vi "Read Shared Variables - SuNLaMP DO.vi"(9 "channel errors in (no errors)":errorcluster[](array[cluster])) -> (1 "channel errors out":errorcluster[](array[cluster]), 2 "data":dbl[](array[numeric]), 3 "UUIDs":string[](array[string])=["Flow Rate [g/s]", "Density [g/cm^3]", "Return Filter dP [psid]", "Outlet Filter and Flowmeter dp [psid]", "Cooler dP [psid]", "Cooler CO2 In [F]", "Cooler CO2 Out [F]", "Pump Frequency [%]", "Recirc Valve Open [%]"])   [LabVIEW 2020]
uses:
  <vilib>/Utility/error.llb/Error Cluster From Error Code.vi
  <vilib>/ErrorRing/Error Ring.xnode
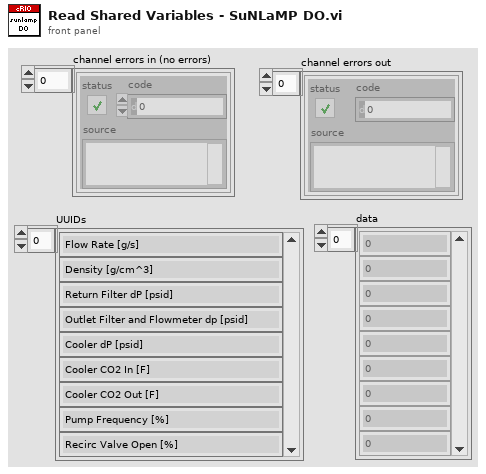
[diagram p1: front panel]
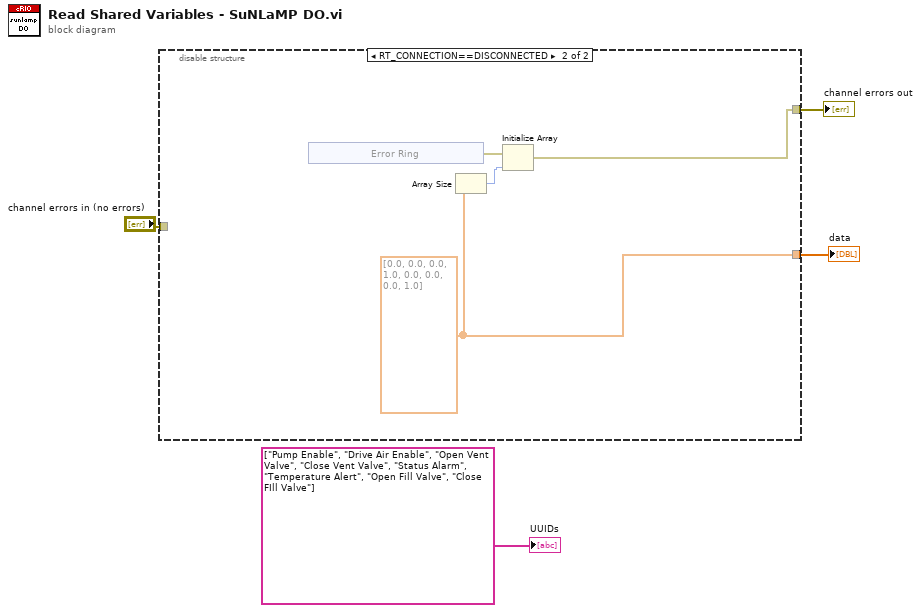
[diagram p0: block diagram]
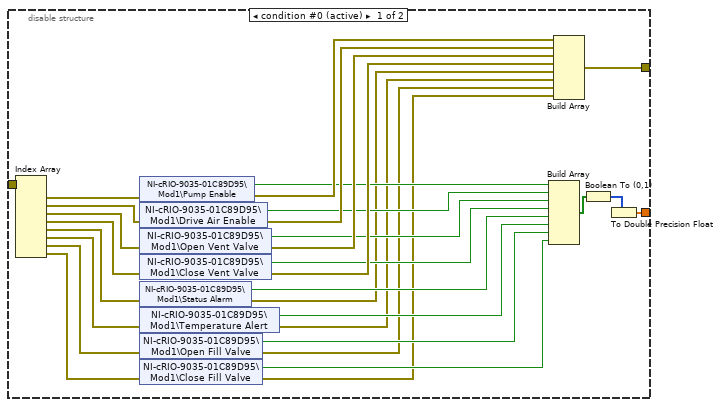
[diagram p2: hidden frame]
diagram:
  n1 = disable-structure shown="RT_CONNECTION==DISCONNECTED" {
    disable-tunnel: [w24 w35] -> w3
    disable-tunnel: "channel errors in (no errors)" -> [w23 _]
    disable-tunnel: [w17 w34] -> w1
    frame condition #0 (active) {
      n2 = Index Array(array=w23) -> (element #1=w22:errorcluster, element #2=w21:errorcluster, element #3=w20:errorcluster, element #4=w19:errorcluster, element #5=w16:errorcluster, element #6=w15:errorcluster, element #7=w14:errorcluster, element #8=w13:errorcluster)  [unwired: 8 in]
      n3 = shared-variable "NI-cRIO-9035-01C89D95\\Mod1\\Pump Enable"(error in=w22) -> (w26:bool, error out=w30:errorcluster)
      n4 = shared-variable "NI-cRIO-9035-01C89D95\\Mod1\\Drive Air Enable"(error in=w21) -> (w27:bool, error out=w31:errorcluster)
      n5 = shared-variable "NI-cRIO-9035-01C89D95\\Mod1\\Open Vent Valve"(error in=w20) -> (w28:bool, error out=w32:errorcluster)
      n6 = shared-variable "NI-cRIO-9035-01C89D95\\Mod1\\Close Vent Valve"(error in=w19) -> (w29:bool, error out=w33:errorcluster)
      n7 = shared-variable "NI-cRIO-9035-01C89D95\\Mod1\\Status Alarm"(error in=w16) -> (w12:bool, error out=w8:errorcluster)
      n8 = shared-variable "NI-cRIO-9035-01C89D95\\Mod1\\Temperature Alert"(error in=w15) -> (w11:bool, error out=w7:errorcluster)
      n9 = shared-variable "NI-cRIO-9035-01C89D95\\Mod1\\Open Fill Valve"(error in=w14) -> (w10:bool, error out=w6:errorcluster)
      n10 = shared-variable "NI-cRIO-9035-01C89D95\\Mod1\\Close Fill Valve"(error in=w13) -> (w9:bool, error out=w5:errorcluster)
      n11 = Build Array(w26, w27, w28, w29, w12, w11, w10, w9) -> (w25:bool[])
      n12 = Build Array(w30, w31, w32, w33, w8, w7, w6, w5) -> (w24:errorcluster[])
      n13 = Boolean To (0,1)(Boolean=w25) -> (0, 1=w18:i16[])
      n14 = To Double Precision Float(number=w18) -> (double precision float=w17:dbl[])
    }
    frame condition #1 {
      w34 = dbl[] [0.0, 0.0, 0.0, 1.0, 0.0, 0.0, 0.0, 1.0] ("data")
      n15 = xnode "Error Ring"() -> ("error out"=w37:errorcluster)
      n16 = Array Size(array=w34) -> (size(s)=w36:i32)
      n17 = Initialize Array(w37, w36) -> (w35:errorcluster[])
    }
  }
  "data" <- w1
  "channel errors out" <- w3
  "UUIDs" <- string[] ["Pump Enable", "Drive Air Enable", "Open Vent Valve", "Close Vent Valve", "Status Alarm", "Temperature Alert", "Open Fill Valve", "Close FIll Valve"]
